vi "PM-P-filter_waveform.vi"(8 "error in (no error)":errorcluster, 11 "loop data":T1) -> (0 "error out":errorcluster, 3 "loop data":T1)   [LabVIEW 2020]
uses:
  PM-P-loop_data.ctl
  PM-P-user_events.ctl
  init-close/PM-common-heartrate_data.ctl
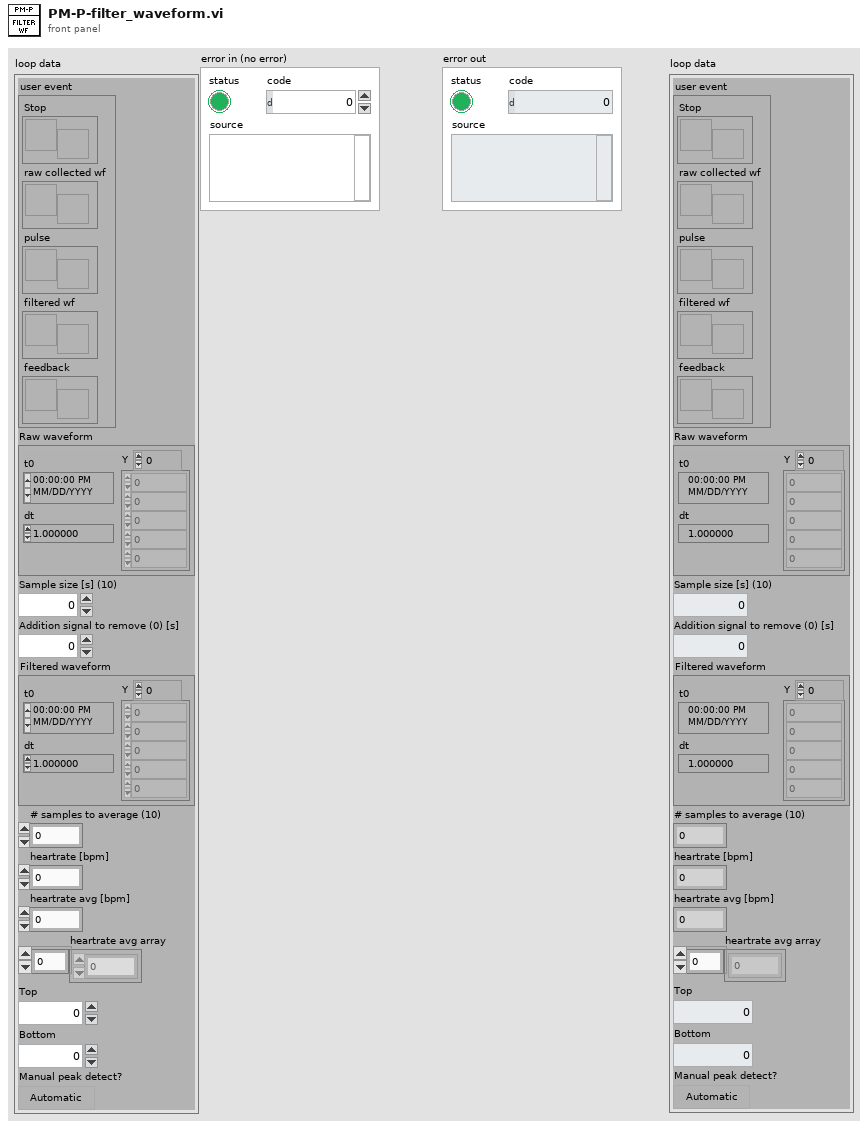
[diagram p1: front panel]
types:
  T1 = typedef "PM-P-loop_data.ctl" = cluster{"user event":T2, "Raw waveform":waveform(dbl), "Sample size [s] (10)":i32, "Addition signal to remove (0) [s]":dbl, "Filtered waveform":waveform(dbl), "# samples to average (10)":i32, "heartrate [bpm]":dbl, "heartrate avg [bpm]":dbl, "heartrate avg array":dbl[], "Top":dbl, "Bottom":dbl, "Manual peak detect?":bool}
  T2 = typedef "PM-P-user_events.ctl" = cluster{"Stop":refnum<user-event>, "raw collected wf":refnum<user-event>, "pulse":refnum<user-event>, "filtered wf":refnum<user-event>, "feedback":refnum<user-event>}
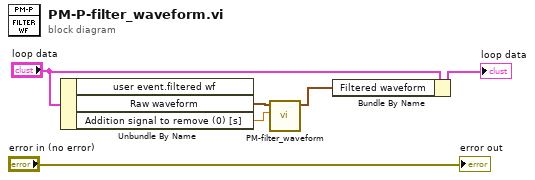
[diagram p0: block diagram]
diagram:
  n1 = Unbundle By Name("loop data") -> ("Raw waveform"=w5:waveform(dbl), "Addition signal to remove (0) [s]"=w4:dbl)  [unwired: 1 out]
  n2 = call "PM-filter_waveform.vi"("Addition signal to remove (0) [s]"=w4, "waveform in"=w5) -> ("waveform out"=w1:waveform(dbl))  [unwired: 8 in, 1 out]
  n3 = Bundle By Name(cluster="loop data", "Filtered waveform"=w1) -> (→"loop data":T1)
  "error out" <- "error in (no error)"
